vi "Quick Stacks - Image Multi Stacks.vi"(7 "Calling VI Ref":refnum<vi>) -> ()   [LabVIEW 2020]
uses:
  <vilib>/Utility/miscctls.llb/LVPointTypeDef.ctl
  Quick Stacks Type Defs/Quick Stack Marked Areas Actions.ctl
  Quick Stacks Type Defs/Quick Stacks Notifier Type.ctl
  Quick Stacks Type Defs/Quick Stack Actions.ctl
  Hardware Configuration/Hardware Configuration Controls/Device Function.ctl
  Hardware Configuration/Hardware Configuration Controls/Device Type.ctl
  Device Library/Stages/Stages Controls/Stage Actions.ctl
  Quick Stacks Type Defs/Quick Stacks Multi Stack Meta Data.ctl
  Device Library/Microscopes/Polymorphic Microscope Messenger/Get Obj Z Pos.vi
  Device Library/Microscopes/Polymorphic Microscope Messenger/Set Obj Z Pos.vi
panel:
  out "Current Delay Time (s)":dbl=1.0 format="%.1f"
  out "Current Cycle":u16=1 min=1
  out "XY Positions":cluster{dbl[], dbl[]}[](graph)
  in  "Cycle Delay (s)":u32
  in  "Number of Cycles":u16=1 min=1
  in  "Capture":bool
  in  "Clear All":bool
  in  "Clear Selected":bool
  in  "Mark Point":bool
  in  "Marked Positions":i32(listbox)
  in  "Quit":bool
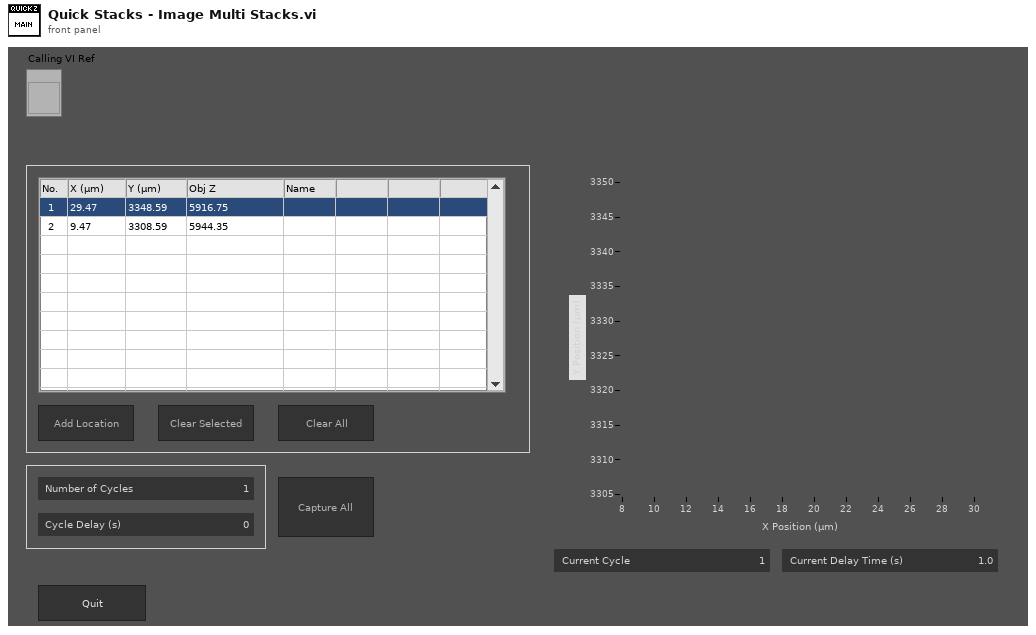
[diagram p1: front panel]
types:
  T1 = typedef "Quick Stacks Notifier Type.ctl" = cluster{"Actions":T2, "Start Z (µm)":dbl, "End Z (µm)":dbl, "Z Size (µm)":dbl, "Num of Steps":u16, "Frames per Step":u16, "Cycle Delay (s)":u32, "Num of Cycles":u16, "Save Path":path, "Running?":bool, "Save File Refs":refnum<file>[]}
  T2 = typedef "Quick Stack Actions.ctl" = enum16{"Idle", "Update Range", "Start Acquisition", "Initial C Step", "Open File", "Close File", "Start Camera", "Stop Camera", "Wait New Frame", "Laser On", "Laser Off", "Get Image", "Step Z", "Move to Z Start", "Step Color", "Check Cycle", "Abort", "Exit Loop", "Quit"}
  T3 = typedef "Quick Stack Marked Areas Actions.ctl" = enum16{"Add Position", "Update File Name", "Remove Position", "Start Capture", "Move to Position", "Write Meta Data", "Capture", "Switch", "Delay", "Reset Path", "Clear All", "Abort", "Exit Loop", "Quit"}
  T4 = enum16{"Always On", "Always Off", "Off While Running"}
  T5 = typedef "LVPointTypeDef.ctl" = cluster{"Horizontal":i16, "Vertical":i16}
  T6 = typedef "Device Function.ctl" = enum16{"Primary", "Secondary", "Overview", "Wide Field Drift Correction", "642 nm Excitation", "560 nm Excitation", "940 nm Excitation", "546 nm Excitation", "488 nm Excitation", "405 nm Excitation", "Objective Drift Correction", "4Pi Objective Lock", "Objective XY", "Objective Z", "Sample XY", "Sample Coarse Z", "Sample Z", "4Pi Lower", "4Pi Upper", "Mojo", "Adj Cavity", "Line Scanning", "Alert"}
  T7 = typedef "Device Type.ctl" = enum16{"AOTF", "Camera", "Deformable Mirror", "Laser", "Microscope Base", "Shutter", "Stage", "Waveform", "FPGA", "Email", "Filter Wheel", "Spinning Disk"}
  T8 = typedef "Stage Actions.ctl" = enum16{"Get Position", "MVR", "MOVE", "HALT", "ONTARGET", "ERROR", "REFERENCE", "INIT", "VELOCITY", "STATUS", "EXIT", "HOME", "ZEROPOS", "NANOPOS", "ANALOG", "QUIT"}
  T9 = typedef "Quick Stacks Multi Stack Meta Data.ctl" = cluster{"Start Z (µm)":dbl, "End Z (µm)":dbl, "Z Size (µm)":dbl, "Num of Steps":u16, "Frames per Step":u16, "Cycle Delay (s)":u32, "Num of Cycles":u16}
  T10 = enum32{"Invalid", "Standard", "Closed", "Hidden", "Minimized", "Maximized"}
  T11 = enum8{"Enabled", "Disabled", "Disabled and Grayed Out"}
  T12 = typedef "LVRectTypeDef.ctl" = cluster{"Left":i16, "Top":i16, "Right":i16, "Bottom":i16}
  T13 = typedef "LVBoundsTypeDef.ctl" = cluster{"Width":u32, "Height":u32}
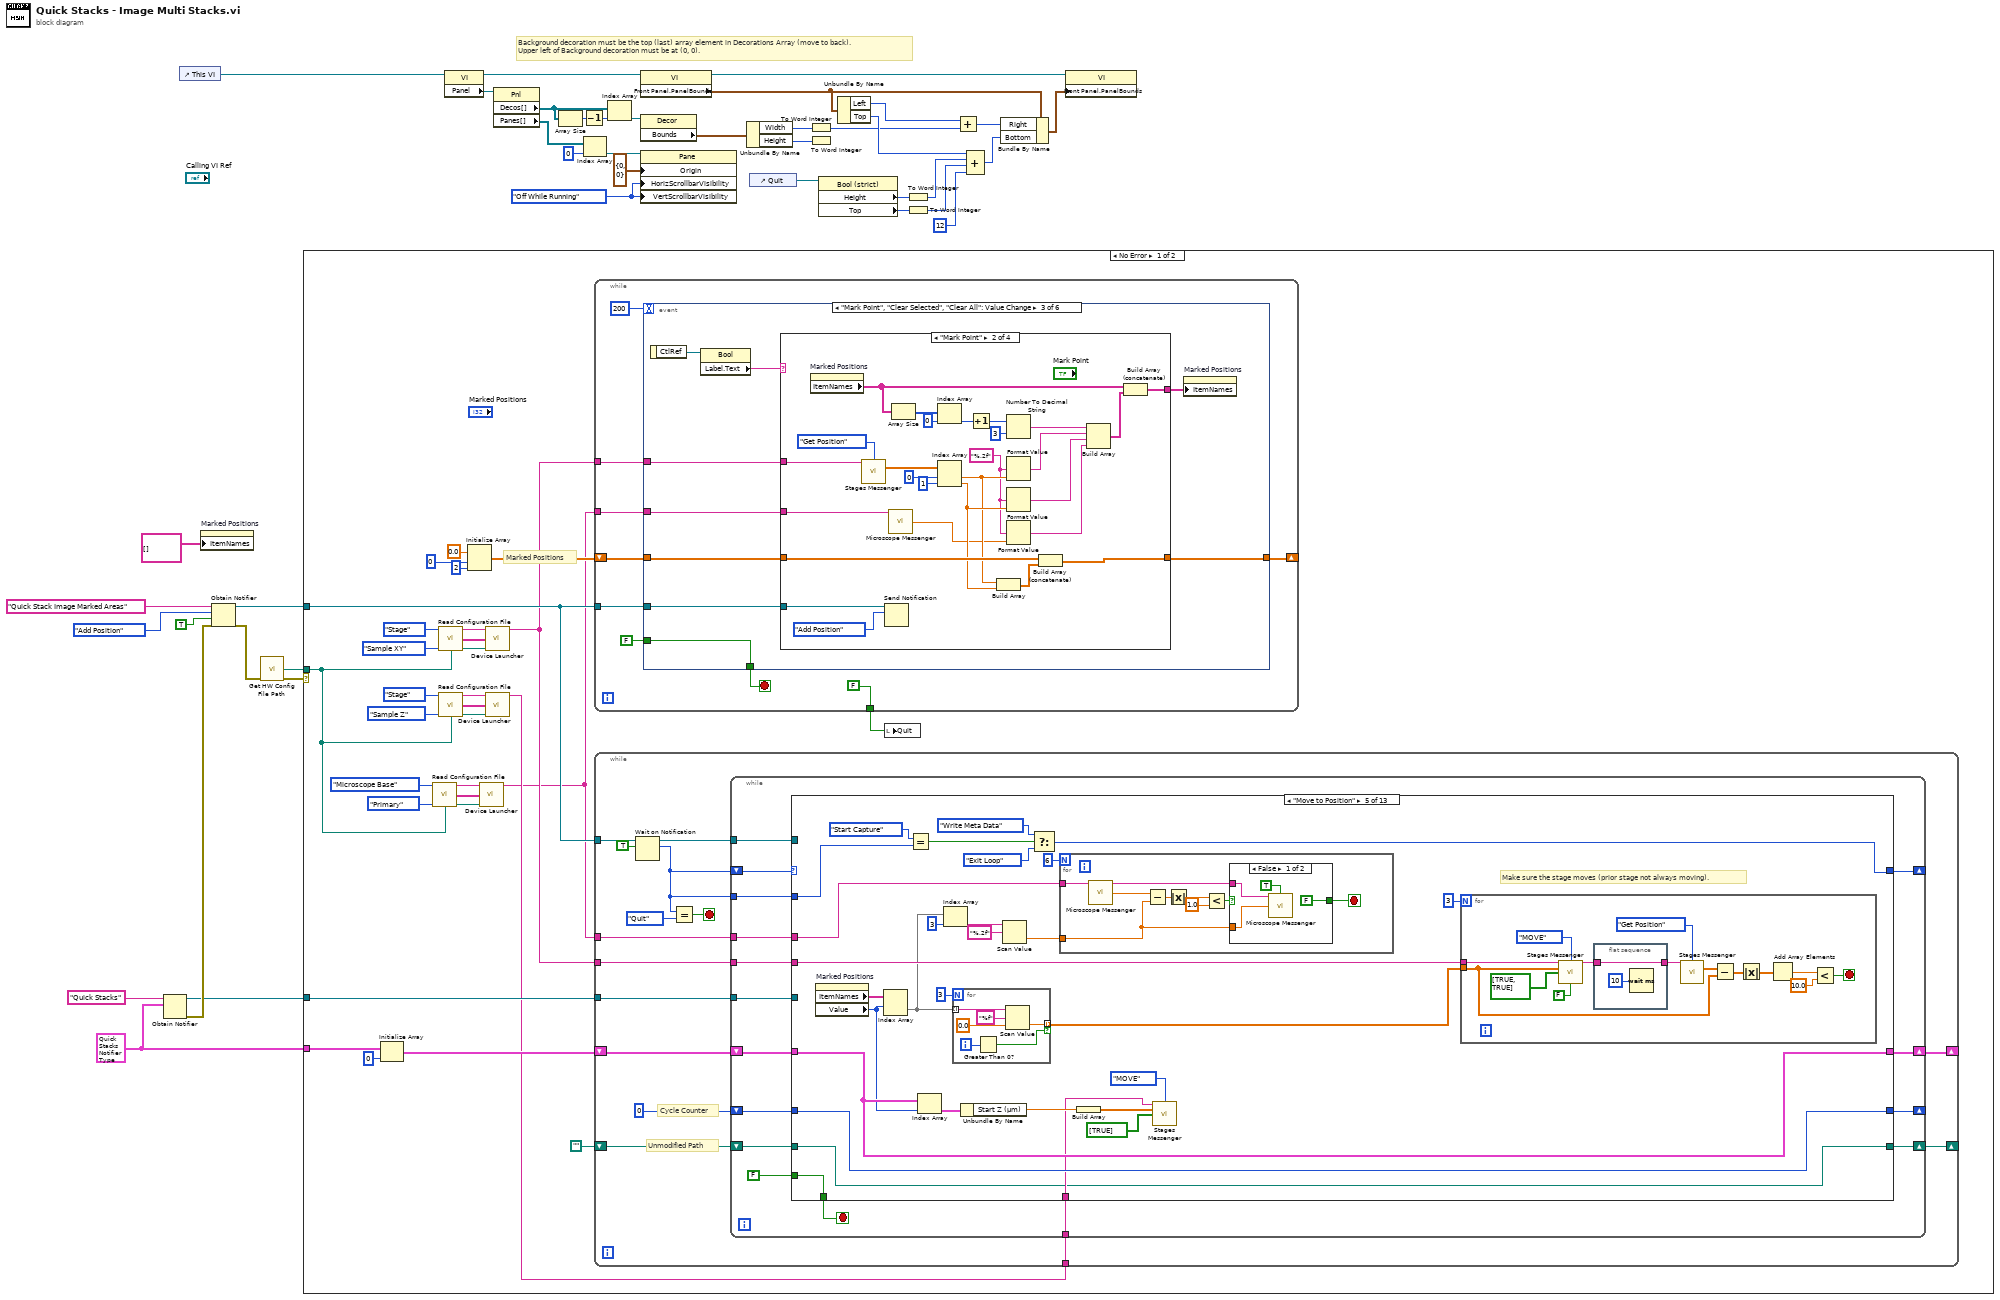
[diagram p0: block diagram]
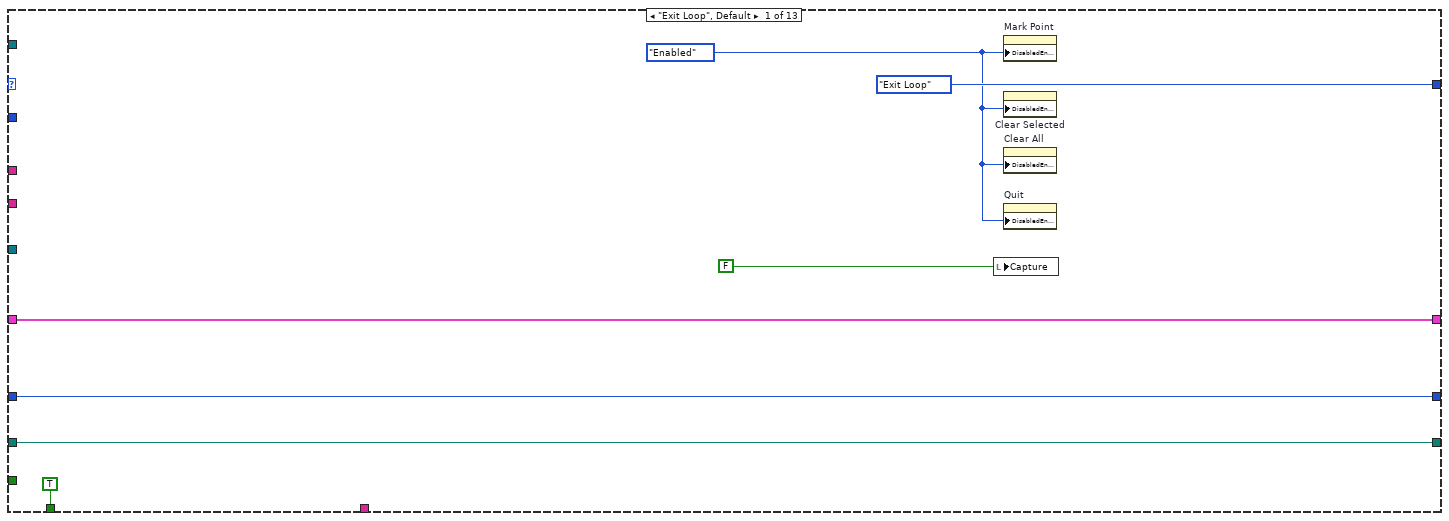
[diagram p2: hidden frame]
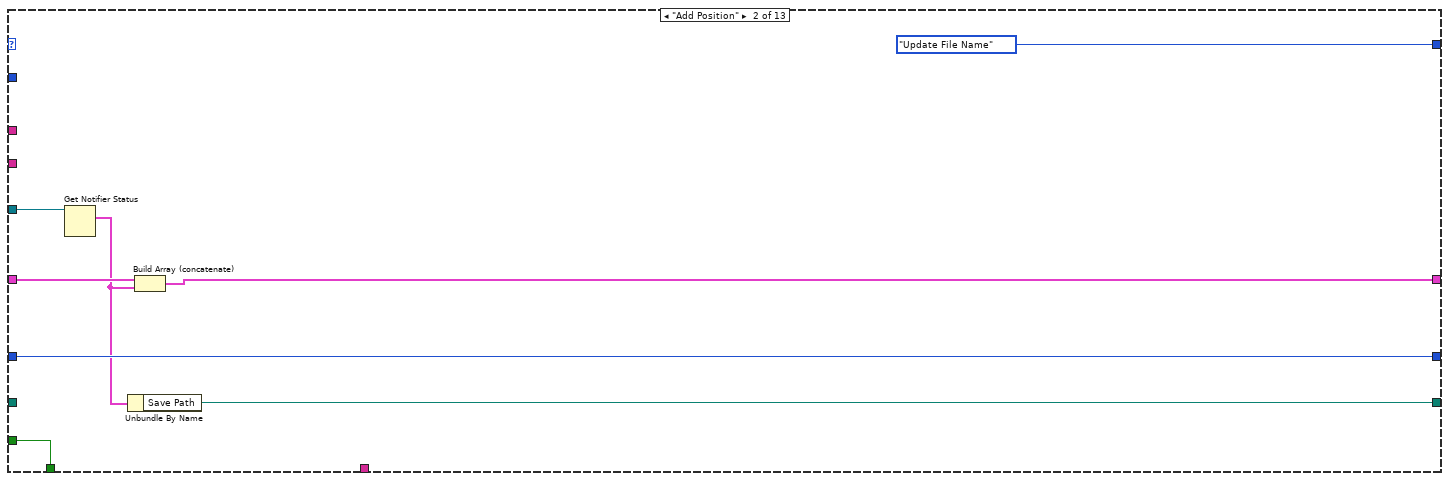
[diagram p3: hidden frame]
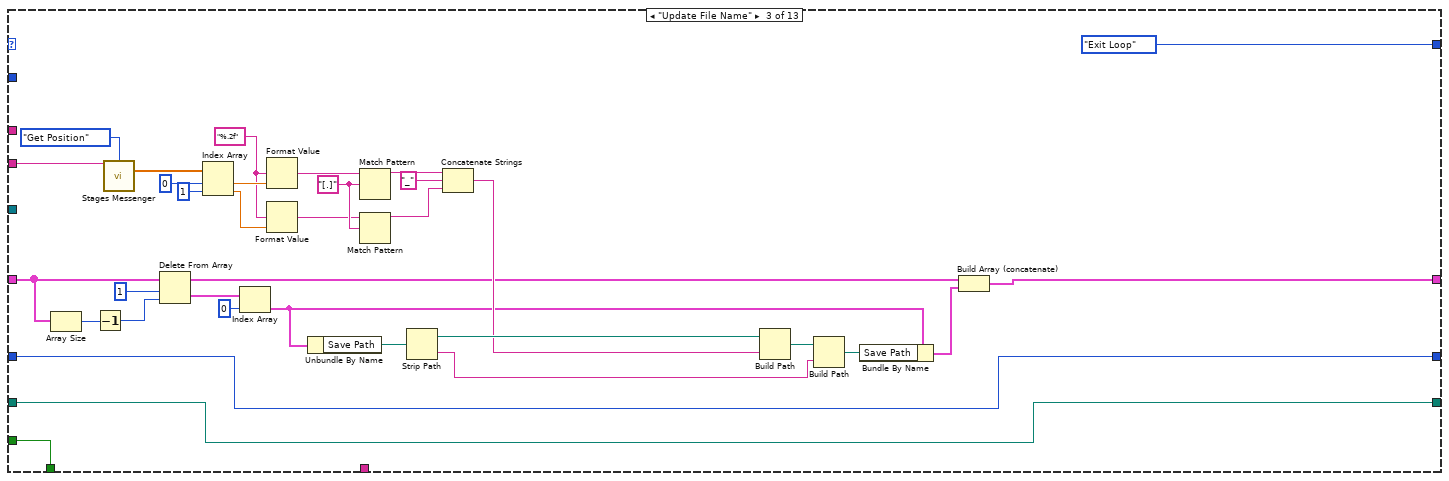
[diagram p4: hidden frame]
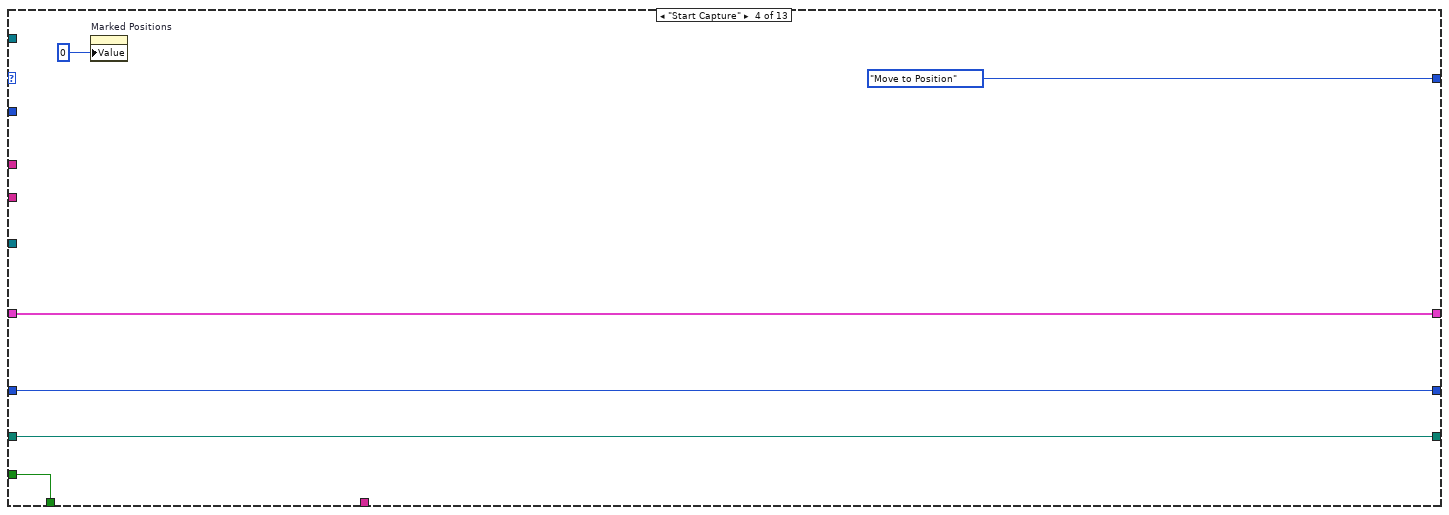
[diagram p5: hidden frame]
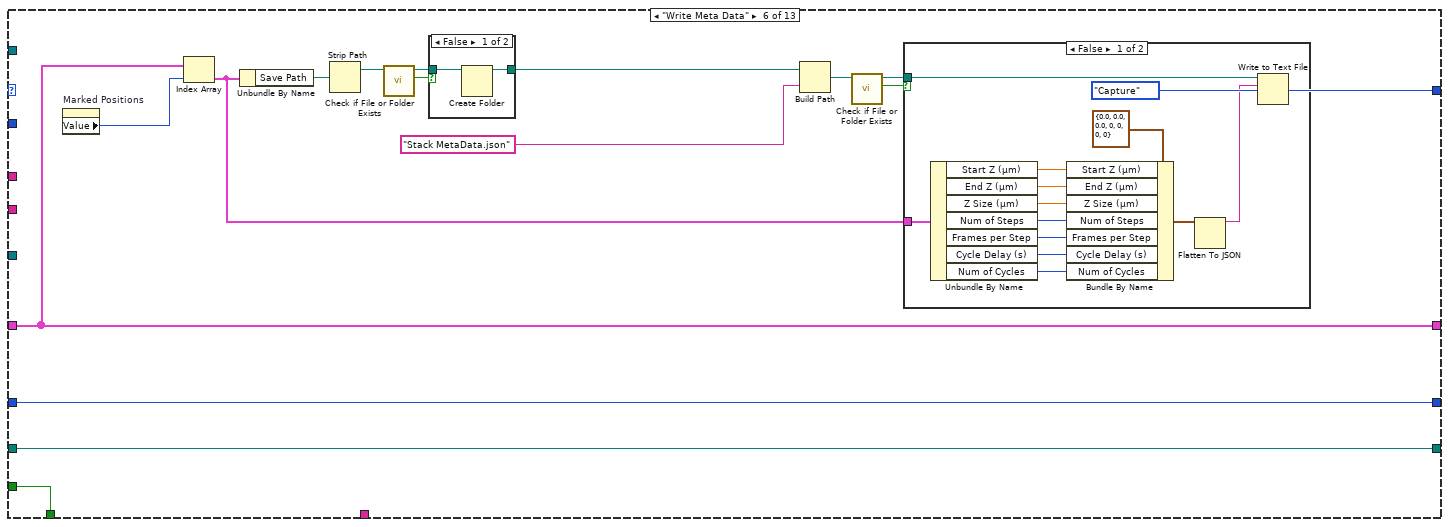
[diagram p7: hidden frame]
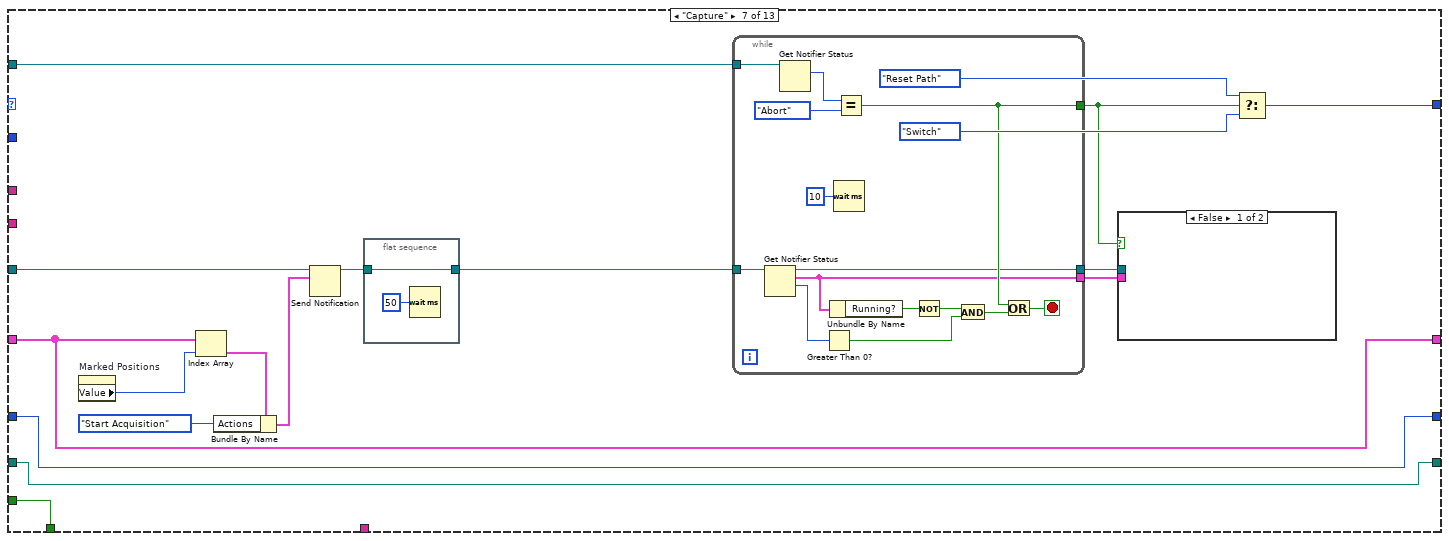
[diagram p10: hidden frame]
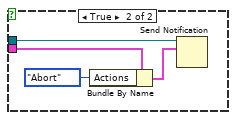
[diagram p11: hidden frame]
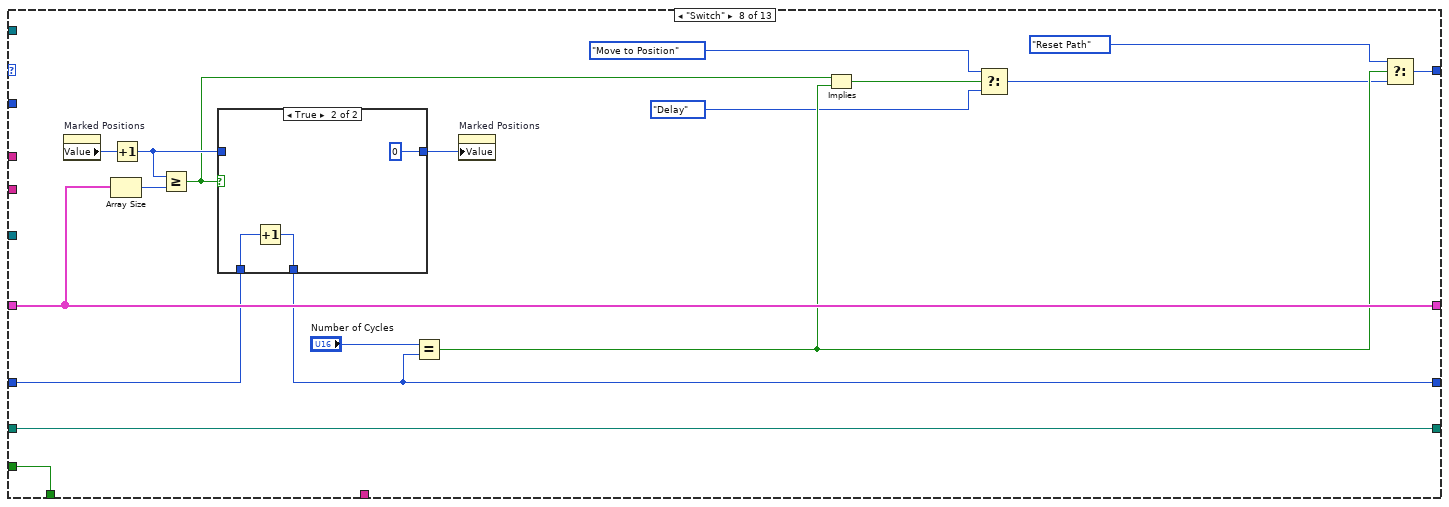
[diagram p12: hidden frame]
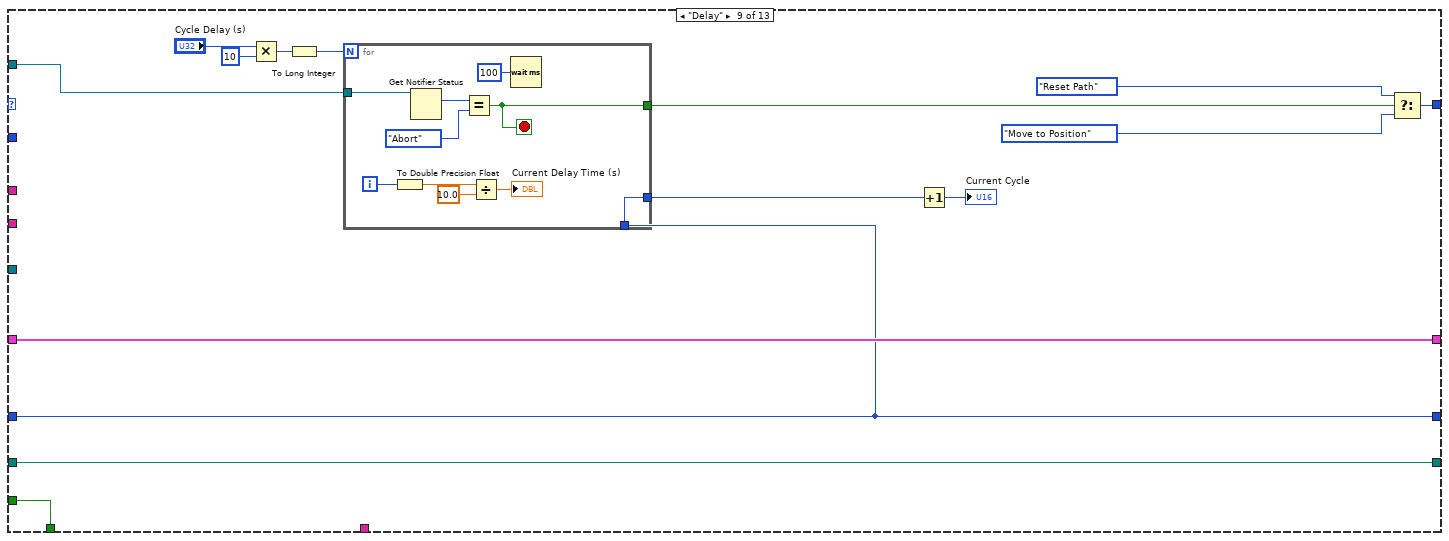
[diagram p14: hidden frame]
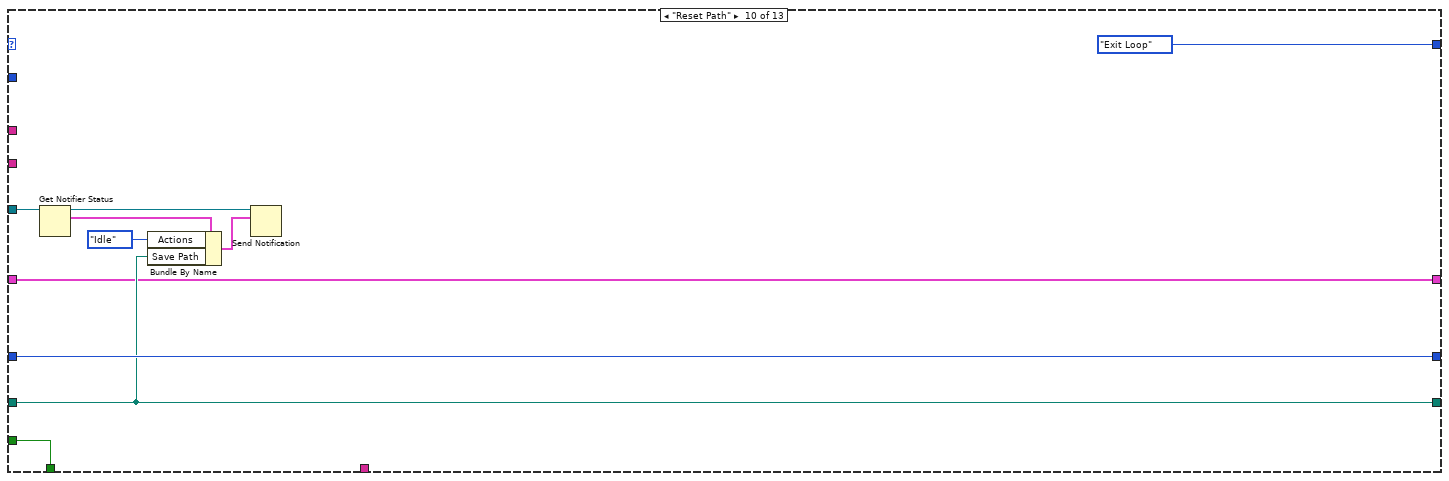
[diagram p15: hidden frame]
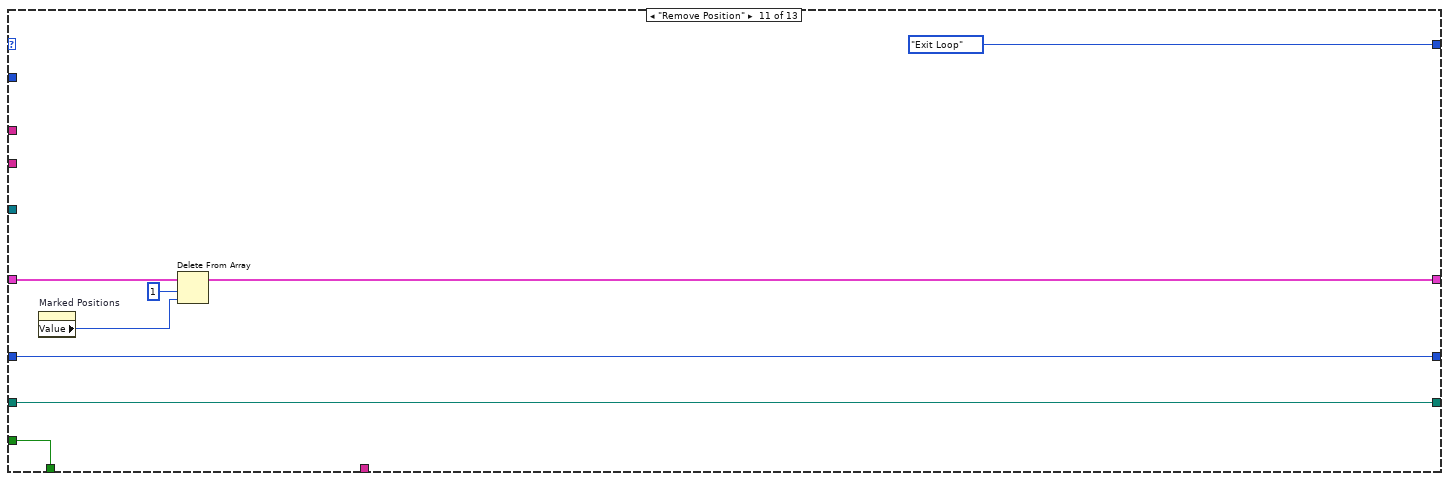
[diagram p16: hidden frame]
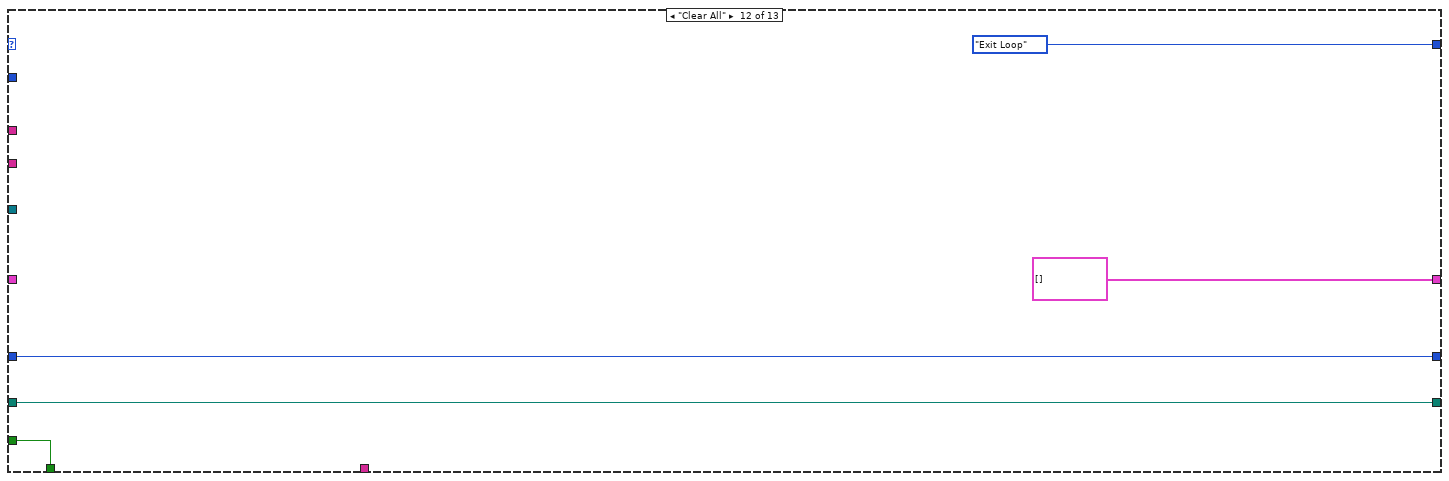
[diagram p17: hidden frame]
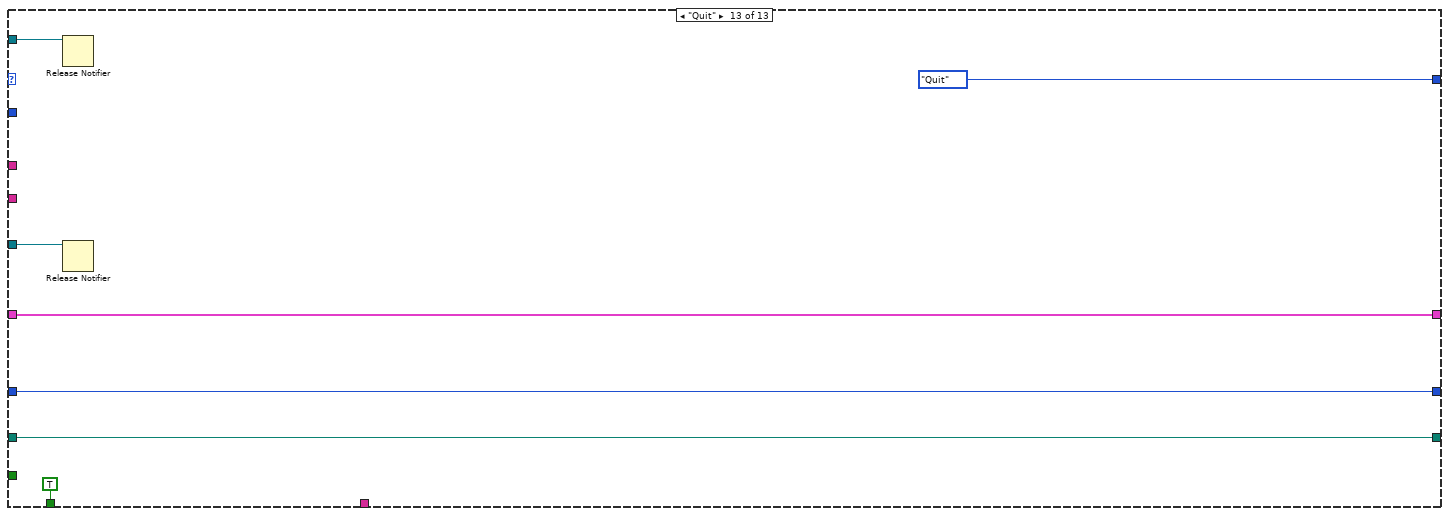
[diagram p18: hidden frame]
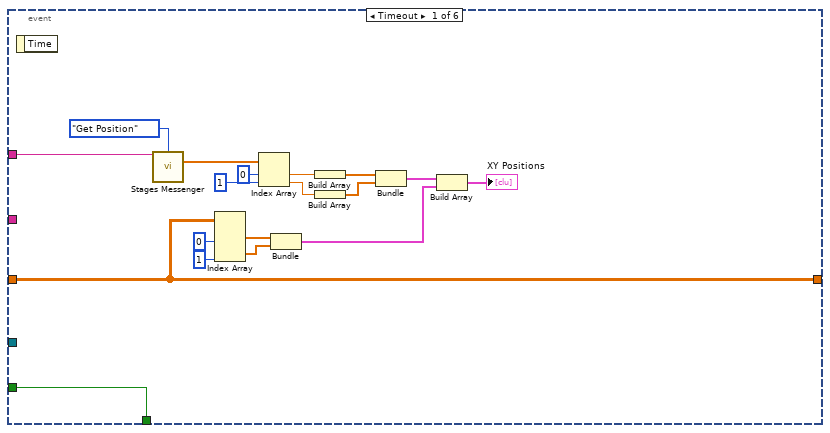
[diagram p19: hidden frame]
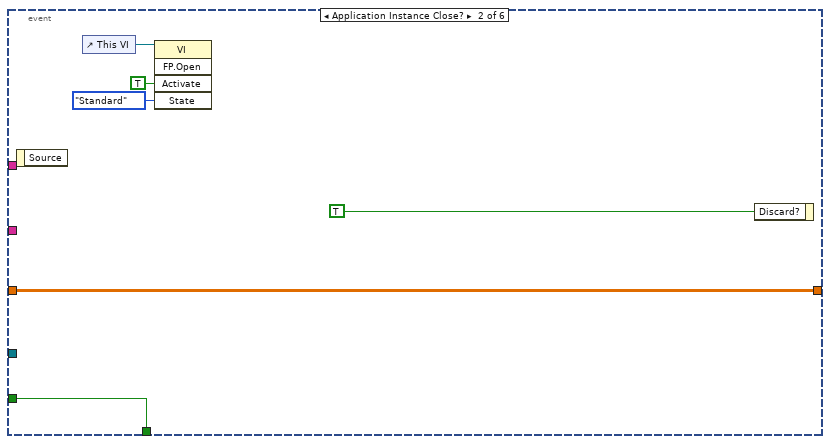
[diagram p20: hidden frame]
diagram:
  w1 = T1 {"Actions"=enum."Idle", "Start Z (µm)"=0.0, "End Z (µm)"=0.0, "Z Size (µm)"=0.0, "Num of Steps"=0, "Frames per Step"=0, "Cycle Delay (s)"=0, "Num of Cycles"=0, "Save Path"=path "", "Running?"=FALSE, "Save File Refs"=[]} ("Stack Parameters")
  w22 = T4."Off While Running" ("Vertical Scrollbar Visibility")
  # "Background decoration must be the top (last) array element in Decorations Array (move to back).\nUpper left of Background decoration must be at (0, 0)."
  n1 = Obtain Notifier(name (unnamed)="Quick Stacks", notification data type=w1) -> (notifier out=w2:refnum<notifier>, error out=w3:errorcluster)  [unwired: 2 in, 1 out]
  n2 = control-ref of="This VI"() -> (w14:refnum<vi>)
  n3 = property on="Marked Positions" class="MCListbox (strict)"("ItemNames"=string[][] [] ("Item Names")) -> ()  [unwired: 2 in, 2 out]
  n4 = Obtain Notifier(name (unnamed)="Quick Stack Image Marked Areas", notification data type=Quick_Stack_Marked_Areas_Actions."Add Position" ("Actions"), create if not found? (T)=TRUE, error in (no error)=w3) -> (notifier out=w7:refnum<notifier>, error out=w8:errorcluster)  [unwired: 1 out]
  n5 = call "Get HW Config File Path.vi"("Error"=w8) -> ("File Path"=w40:path, "Error"=w41:errorcluster)  [unwired: 13 in]
  n6 = case shown="No Error" w41 {
    tunnel: w40 -> [w43 _]
    tunnel: w7 -> [w65 _]
    tunnel: w2 -> [w63 _]
    tunnel: w1 -> [w62 _]
    frame No Error {
      # "Marked Positions"
      n7 = Initialize Array(w62, 0 ("dimension size")) -> (w60:T1[])
      n8 = call "Read Configuration File.vi"("Device Type"=Device_Type."Microscope Base", "Device Function"=Device_Function."Primary", "Config File Path"=w43) -> ("Unique Notifier Name"=w46:string, "Device Ports/IDs/Channels"=w48:string[], "Device Engine Path"=w47:path)  [unwired: 9 in, 1 out]
      n9 = call "Read Configuration File.vi"("Device Type"=Device_Type."Stage", "Device Function"=Device_Function."Sample XY", "Config File Path"=w43) -> ("Unique Notifier Name"=w69:string, "Device Ports/IDs/Channels"=w71:string[], "Device Engine Path"=w70:path)  [unwired: 9 in, 1 out]
      n10 = call "Read Configuration File.vi"("Device Type"=Device_Type."Stage", "Device Function"=Device_Function."Sample Z", "Config File Path"=w43) -> ("Unique Notifier Name"=w53:string, "Device Ports/IDs/Channels"=w51:string[], "Device Engine Path"=w52:path)  [unwired: 9 in, 1 out]
      n11 = Initialize Array(0.0 ("element"), 0 ("dimension size"), 2 ("dimension size")) -> (w58:dbl[][])
      n12 = call "Device Launcher.vi"("Notifier Name"=w46, "Device Ports/IDs/Channels"=w48, "Device Engine Path"=w47) -> ("Notifier Name"=w42:string)  [unwired: 11 in, 1 out]
      n13 = call "Device Launcher.vi"("Notifier Name"=w69, "Device Ports/IDs/Channels"=w71, "Device Engine Path"=w70) -> ("Notifier Name"=w64:string)  [unwired: 11 in, 1 out]
      n14 = call "Device Launcher.vi"("Notifier Name"=w53, "Device Ports/IDs/Channels"=w51, "Device Engine Path"=w52) -> ("Notifier Name"=w50:string)  [unwired: 11 in, 1 out]
      n15 = while {
        tunnel: [FALSE] -> w66
        tunnel: w64 -> [w374]
        tunnel: w65 -> [w373]
        shift-right: [w371] -> _
        shift-left: w58 -> [w372]
        tunnel: w42 -> [w370]
        stop <- w376 stop-if-true
        n16 = event shown="[2] \"Mark Point\", \"Clear Selected\", \"Clear All\": Value Change" {
          selector: _ -> [_ _ _ _ _ _]
          dyn-events: _ -> [_ _ _ _ _ _]
          timeout: 200 -> [_ _ _ _ _ _]
          tunnel: FALSE -> [w396 w401 w411 w466 w476 _]
          tunnel: [w396 w401 w411 w466 w476 w480] -> w376
          tunnel: w374 -> [w394 _ w408 _ _ _]
          tunnel: w373 -> [_ _ w406 w465 w475 w479]
          tunnel: w372 -> [w386 w397 w405 w463 w467 w477]
          tunnel: [w386 w397 w404 w463 w467 w477] -> w371
          tunnel: w370 -> [_ _ w403 _ _ _]
          event Timeout {
            n17 = event-data() -> ()  [unwired: 1 in, 1 out]
            n18 = call "Stages Messenger.vi"("Stage Notifier Name"=w394, "Actions"=Stage_Actions."Get Position") -> ("Positions"=w393:dbl[])  [unwired: 10 in, 3 out]
            n19 = Index Array(array=w386, index (col) #1=0 ("disabled index (col)"), index (col) #2=1 ("index (col)")) -> (element #1=w383:dbl[], element #2=w382:dbl[])  [unwired: 2 in]
            n20 = Index Array(array=w393, index #1=0 ("index"), index #2=1 ("index")) -> (element #1=w390:dbl, element #2=w389:dbl)
            n21 = Bundle(w383, w382) -> (w380:cluster{dbl[], dbl[]})  [unwired: 1 in]
            n22 = Build Array(w390) -> (w388:dbl[])
            n23 = Build Array(w389) -> (w387:dbl[])
            n24 = Bundle(w388, w387) -> (w381:cluster{dbl[], dbl[]})  [unwired: 1 in]
            n25 = Build Array(w381, w380) -> (→"XY Positions":cluster{dbl[], dbl[]}[])
          }
          event Application Instance Close? {
            n26 = event-data() -> ()  [unwired: 1 in, 1 out]
            n27 = control-ref of="This VI"() -> (w398:refnum<vi>)
            n28 = invoke class="VI" method="FP.Open"(reference=w398, "Activate"=TRUE ("Activate?"), "State"=T10."Standard") -> ()  [unwired: 2 in, 5 out]
            n29 = event-data("Discard?"=TRUE) -> ()  [unwired: 1 in, 1 out]
          }
          event "Mark Point", "Clear Selected", "Clear All": Value Change {
            n30 = event-data() -> ("CtlRef"=w410:refnum<vi>)  [unwired: 1 in]
            n31 = property class="Bool"(reference=w410) -> ("Label.Text"=w407:string)  [unwired: 1 in, 2 out]
            n32 = case shown="\"Mark Point\"" w407 {
              tunnel: [w415 w431 w452 string[][] []] -> w409
              tunnel: w408 -> [_ w429 _ _]
              tunnel: w406 -> [w414 w428 w450 w461]
              tunnel: w405 -> [w412 w426 w446 _]
              tunnel: [w412 w422 w444 w456] -> w404
              tunnel: w403 -> [_ w421 _ _]
              frame Default {
                n33 = Send Notification(notification=Quick_Stack_Marked_Areas_Actions."Exit Loop", notifier=w414) -> ()  [unwired: 1 in, 2 out]
                n34 = property on="Marked Positions" class="MCListbox (strict)"() -> ("ItemNames"=w415:string[][])  [unwired: 2 in, 2 out]
              }
              frame "Mark Point" {
                w419 = "%.2f" ("format string")
                n35 = property on="Marked Positions" class="MCListbox (strict)"() -> ("ItemNames"=w418:string[][])  [unwired: 2 in, 2 out]
                n36 = call "Stages Messenger.vi"("Stage Notifier Name"=w429, "Actions"=Stage_Actions."Get Position") -> ("Positions"=w430:dbl[])  [unwired: 10 in, 3 out]
                n37 = Send Notification(notification=Quick_Stack_Marked_Areas_Actions."Add Position", notifier=w428) -> ()  [unwired: 1 in, 2 out]
                n38 = call-poly "Microscope Messenger.vi"("Notifier Name In"=w421) -> ("Obj Z Pos"=w416:dbl)  [unwired: 12 in, 2 out]
                n39 = Array Size(array=w418) -> (size(s)=w437:i32[])
                n40 = Index Array(array=w437, index=0) -> (element=w435:i32)
                n41 = Index Array(array=w430, index #1=0 ("index"), index #2=1 ("index")) -> (element #1=w424:dbl, element #2=w425:dbl)
                n42 = Increment(x=w435) -> (x+1=w439:i32)
                n43 = Build Array(w424, w425) -> (w423:dbl[])
                n44 = Number To Decimal String(number=w439, width (-)=i16 3) -> (decimal integer string=w434:string)
                n45 = Format Value(format string=w419, value (0)=w424) -> (output string=w433:string)  [unwired: 1 in]
                n46 = Format Value(format string=w419, value (0)=w425) -> (output string=w420:string)  [unwired: 1 in]
                n47 = Format Value(format string=w419, value (0)=w416) -> (output string=w417:string)  [unwired: 1 in]
                n48 = Build Array (concatenate)(w426, w423) -> (w422:dbl[][])
                n49 = Build Array(w434, w433, w420, w417) -> (w432:string[])
                n50 = Build Array (concatenate)(w418, w432) -> (w431:string[][])
              }
              frame "Clear Selected" {
                n51 = Send Notification(notification=Quick_Stack_Marked_Areas_Actions."Remove Position", notifier=w450) -> (error out=w448:errorcluster)  [unwired: 1 in, 1 out]
                n52 = flat-sequence {
                  tunnel: w448 -> [w454]
                  tunnel: [w454] -> w447
                  frame #0 {
                    n53 = Wait (ms)(milliseconds to wait=u32 10) -> ()  [unwired: 1 out]
                  }
                }
                n54 = property on="Marked Positions" class="MCListbox (strict)"() -> ("ItemNames"=w453:string[][])  [unwired: 2 in, 2 out]
                n55 = property on="Marked Positions" class="MCListbox (strict)"(error in=w447) -> ("Value"=w445:i32)  [unwired: 1 in, 2 out]
                n56 = Delete From Array(array=w453, length=1, index (row)=w445) -> (array with subset deleted=w452:string[][])  [unwired: 1 in, 1 out]
                n57 = Delete From Array(array=w446, length=1, index (row)=w445) -> (array with subset deleted=w444:dbl[][])  [unwired: 1 in, 1 out]
              }
              frame "Clear All" {
                n58 = Send Notification(notification=Quick_Stack_Marked_Areas_Actions."Clear All", notifier=w461) -> ()  [unwired: 1 in, 2 out]
                n59 = Initialize Array(0.0 ("element"), 0 ("dimension size"), 2 ("dimension size")) -> (w456:dbl[][])
              }
            }
            n60 = property on="Marked Positions" class="MCListbox (strict)"("ItemNames"=w409) -> ()  [unwired: 2 in, 2 out]
          }
          event "Marked Positions": Double Click {
            n61 = event-data() -> ()  [unwired: 1 in, 1 out]
            n62 = Send Notification(notification=Quick_Stack_Marked_Areas_Actions."Move to Position", notifier=w465) -> ()  [unwired: 1 in, 2 out]
          }
          event "Capture": Value Change {
            n63 = event-data() -> ("NewVal"=w472:bool)  [unwired: 1 in]
            n64 = Select(t=Quick_Stack_Marked_Areas_Actions."Start Capture", s=w472, f=Quick_Stack_Marked_Areas_Actions."Abort" ("y")) -> (s? t:f=w473:T3)
            n65 = Select(t=T11."Disabled and Grayed Out" ("Disabled"), s=w472, f=T11."Enabled" ("Disabled")) -> (s? t:f=w469:T11)
            n66 = Send Notification(notification=w473, notifier=w475) -> ()  [unwired: 1 in, 2 out]
            n67 = property on="Mark Point" class="Bool"("DisabledEnum"=w469) -> ()  [unwired: 2 in, 2 out]
            n68 = property on="Clear Selected" class="Bool"("DisabledEnum"=w469) -> ()  [unwired: 2 in, 2 out]
            n69 = property on="Clear All" class="Bool"("DisabledEnum"=w469) -> ()  [unwired: 2 in, 2 out]
            n70 = property on="Quit" class="Bool (strict)"("DisabledEnum"=w469) -> ()  [unwired: 2 in, 2 out]
          }
          event "Quit": Value Change {
            n71 = event-data() -> ("NewVal"=w480:bool)  [unwired: 1 in]
            n72 = Send Notification(notification=Quick_Stack_Marked_Areas_Actions."Quit", notifier=w479) -> ()  [unwired: 1 in, 2 out]
          }
        }
      }
      n73 = while {
        tunnel: w65 -> [w86]
        tunnel: w64 -> [w80]
        tunnel: w63 -> [w79]
        shift-right: [w77] -> _
        shift-left: w60 -> [w78]
        tunnel: w50 -> [w75]
        shift-right: [w74] -> _
        shift-left: path "" -> [w73]
        tunnel: w42 -> [w72]
        stop <- w83 stop-if-true
        # "Unmodified Path"
        # "Cycle Counter"
        n74 = Wait on Notification(notifier=w86, ignore previous (F)=TRUE) -> (notifier out=w82:refnum<notifier>, notification=w81:T3)  [unwired: 2 in, 2 out]
        n75 = Equal?(x=w81, y=Quick_Stack_Marked_Areas_Actions."Quit") -> (x = y?=w83:bool)
        n76 = while {
          shift-right: [w98] -> _
          shift-left: w81 -> [w101]
          tunnel: w82 -> [w102]
          tunnel: w81 -> [w97]
          tunnel: w80 -> [w96]
          tunnel: w79 -> [w95]
          shift-right: [w93] -> w77
          shift-left: w78 -> [w94]
          shift-right: [w91] -> _
          shift-left: u16 0 -> [w92]
          tunnel: w75 -> [w90]
          shift-right: [w89] -> w74
          shift-left: w73 -> [w88]
          tunnel: w72 -> [w87]
          stop <- w99 stop-if-true
          n77 = case shown="\"Move to Position\"" w101 {
            tunnel: w102 -> [_ _ _ _ _ _ w270 _ w320 _ _ _ w367]
            tunnel: [TRUE w117 w151 w157 w186 w237 w271 w309 w329 w348 w356 w361 TRUE] -> w99
            tunnel: FALSE -> [_ w117 w151 w157 w186 w237 w271 w309 w329 w348 w356 w361 _]
            tunnel: [Quick_Stack_Marked_Areas_Actions."Exit Loop" ("y") Quick_Stack_Marked_Areas_Actions."Update File Name" ("y") Quick_Stack_Marked_Areas_Actions."Exit Loop" ("y") Quick_Stack_Marked_Areas_Actions."Move to Position" ("y") w180 Quick_Stack_Marked_Areas_Actions."Capture" ("y") w268 w305 w321 Quick_Stack_Marked_Areas_Actions."Exit Loop" ("y") Quick_Stack_Marked_Areas_Actions."Exit Loop" ("y") Quick_Stack_Marked_Areas_Actions."Exit Loop" ("y") Quick_Stack_Marked_Areas_Actions."Quit" ("y")] -> w98
            tunnel: w97 -> [_ _ _ _ w183 _ _ _ _ _ _ _ _]
            tunnel: w96 -> [_ _ w131 _ w178 _ _ _ _ _ _ _ _]
            tunnel: w95 -> [_ w115 _ _ _ _ w263 _ _ w346 _ _ w366]
            tunnel: w94 -> [w105 w114 w140 w154 w174 w225 w260 w304 w328 w340 w353 _ w365]
            tunnel: [w105 w113 w122 w154 w174 w225 w260 w304 w328 w340 w352 T1[] [] w365] -> w93
            tunnel: w92 -> [w104 w112 w147 w153 w175 w236 w256 w301 w318 w349 w351 w359 w364]
            tunnel: [w104 w112 w147 w153 w175 w236 w256 w299 w318 w349 w351 w359 w364] -> w91
            tunnel: w90 -> [_ _ _ _ w167 _ _ _ _ _ _ _ _]
            tunnel: [w103 w110 w118 w152 w166 w223 w254 w292 w315 w341 w350 w358 w363] -> w89
            tunnel: w88 -> [w103 _ w118 w152 w166 w223 w254 w292 w315 w341 w350 w358 w363]
            tunnel: w87 -> [_ _ _ _ w160 _ _ _ _ _ _ _ _]
            frame "Exit Loop", Default {
              w107 = T11."Enabled" ("Disabled")
              n78 = local write "Capture"(FALSE ("Capture")) -> ()
              n79 = property on="Mark Point" class="Bool"("DisabledEnum"=w107) -> ()  [unwired: 2 in, 2 out]
              n80 = property on="Clear Selected" class="Bool"("DisabledEnum"=w107) -> ()  [unwired: 2 in, 2 out]
              n81 = property on="Clear All" class="Bool"("DisabledEnum"=w107) -> ()  [unwired: 2 in, 2 out]
              n82 = property on="Quit" class="Bool (strict)"("DisabledEnum"=w107) -> ()  [unwired: 2 in, 2 out]
            }
            frame "Add Position" {
              n83 = Get Notifier Status(notifier=w115) -> (current notification=w111:T1)  [unwired: 1 in, 4 out]
              n84 = Unbundle By Name(w111) -> ("Save Path"=w110:path)
              n85 = Build Array (concatenate)(w114, w111) -> (w113:T1[])
            }
            frame "Update File Name" {
              w132 = "%.2f" ("format string")
              w146 = "[.]" ("regular expression")
              n86 = Array Size(array=w140) -> (size(s)=w141:i32)
              n87 = Decrement(x=w141) -> (x-1=w138:i32)
              n88 = call "Stages Messenger.vi"("Stage Notifier Name"=w131, "Actions"=Stage_Actions."Get Position") -> ("Positions"=w133:dbl[])  [unwired: 10 in, 3 out]
              n89 = Delete From Array(array=w140, length=1, index=w138) -> (deleted portion=w126:T1[], array with subset deleted=w127:T1[])
              n90 = Index Array(array=w133, index #1=0 ("index"), index #2=1 ("index")) -> (element #1=w135:dbl, element #2=w134:dbl)
              n91 = Index Array(array=w126, index=0) -> (element=w124:T1)
              n92 = Format Value(format string=w132, value (0)=w135) -> (output string=w129:string)  [unwired: 1 in]
              n93 = Format Value(format string=w132, value (0)=w134) -> (output string=w128:string)  [unwired: 1 in]
              n94 = Unbundle By Name(w124) -> ("Save Path"=w150:path)
              n95 = Match Pattern(string=w129, regular expression=w146) -> (before substring=w145:string)  [unwired: 1 in, 3 out]
              n96 = Match Pattern(string=w128, regular expression=w146) -> (before substring=w144:string)  [unwired: 1 in, 3 out]
              n97 = Strip Path(path=w150) -> (stripped path=w149:path, name=w120:string)
              n98 = Concatenate Strings(w145, "_" ("string"), w144) -> (w142:string)
              n99 = Build Path(base path=w149, name or relative path=w142) -> (appended path=w121:path)
              n100 = Build Path(base path=w121, name or relative path=w120) -> (appended path=w119:path)
              n101 = Bundle By Name(cluster=w124, "Save Path"=w119) -> (w123:T1)
              n102 = Build Array (concatenate)(w127, w123) -> (w122:T1[])
            }
            frame "Start Capture" {
              n103 = property on="Marked Positions" class="MCListbox (strict)"("Value"=0 ("Focus Row")) -> ()  [unwired: 2 in, 2 out]
            }
            frame "Move to Position" {
              # "Make sure the stage moves (prior stage not always moving)."
              n104 = property on="Marked Positions" class="MCListbox (strict)"() -> ("ItemNames"=w179:string[][], "Value"=w173:i32)  [unwired: 2 in, 2 out]
              n105 = Index Array(array=w179, index (row)=w173) -> (element=w164:string[])  [unwired: 1 in]
              n106 = Equal?(x=Quick_Stack_Marked_Areas_Actions."Start Capture" ("y"), y=w183) -> (x = y?=w185:bool)
              n107 = Index Array(array=w174, index=w173) -> (element=w172:T1)
              n108 = Index Array(array=w164, index=3) -> (element=w161:string)
              n109 = for {
                N: 3 -> [_]
                tunnel: w164 -> [w220] mode=indexing
                tunnel: [w219] -> w177 mode=indexing if=w217
                i -> [w218]
                n110 = Greater Than 0?(x=w218) -> (x > 0?=w217:bool)
                n111 = Scan Value(string=w220, format string="%f", default (0 dbl)=0.0) -> (value=w219:dbl)  [unwired: 1 out]
              }
              n112 = Unbundle By Name(w172) -> ("Start Z (µm)"=w170:dbl)
              n113 = Scan Value(string=w161, format string="%.2f") -> (value=w159:dbl)  [unwired: 1 in, 1 out]
              n114 = Select(t=Quick_Stack_Marked_Areas_Actions."Write Meta Data", s=w185, f=Quick_Stack_Marked_Areas_Actions."Exit Loop" ("y")) -> (s? t:f=w180:T3)
              n115 = for {
                N: 6 -> [_]
                tunnel: w160 -> [w195]
                tunnel: w159 -> [w188]
                stop <- w187 stop-if-true
                n116 = call-poly "Microscope Messenger.vi"("Notifier Name In"=w195) -> ("Notifier Name Out"=w192:string, "Obj Z Pos"=w194:dbl)  [unwired: 12 in, 1 out]
                n117 = Subtract(x=w194, y=w188) -> (x-y=w190:dbl)
                n118 = Absolute Value(x=w190) -> (abs(x)=w189:dbl)
                n119 = Less?(x=w189, y=1.0) -> (x < y?=w191:bool)
                n120 = case shown="False" w191 {
                  selector: w191 -> [_ w200]
                  tunnel: w192 -> [w198 _]
                  tunnel: w188 -> [w197 _]
                  tunnel: [FALSE w200] -> w187
                  frame False {
                    n121 = call-poly "Microscope Messenger.vi"("Notifier Name In"=w198, "Wait to Finish"=TRUE, "Obj Z Pos (um)"=w197) -> ()  [unwired: 11 in, 2 out]
                  }
                  frame True {
                  }
                }
              }
              n122 = Build Array(w170) -> (w169:dbl[])
              n123 = call "Stages Messenger.vi"("Stage Notifier Name"=w167, "Actions"=Stage_Actions."MOVE", "Setpoint"=w169, "Axis"=bool[] [TRUE]) -> ()  [unwired: 8 in, 4 out]
              n124 = for {
                N: 3 -> [_]
                tunnel: w178 -> [w211]
                tunnel: w177 -> [w206]
                stop <- w201 stop-if-true
                n125 = call "Stages Messenger.vi"("Stage Notifier Name"=w211, "Actions"=Stage_Actions."MOVE", "Setpoint"=w206, "Axis"=bool[] [TRUE, TRUE], "Exit While Busy?"=FALSE ("Wait for On Target? (F)")) -> ("Stage Notifier Name (Dup)"=w210:string)  [unwired: 7 in, 3 out]
                n126 = flat-sequence {
                  tunnel: w210 -> [w215]
                  tunnel: [w215] -> w208
                  frame #0 {
                    n127 = Wait (ms)(milliseconds to wait=u32 10) -> ()  [unwired: 1 out]
                  }
                }
                n128 = call "Stages Messenger.vi"("Stage Notifier Name"=w208, "Actions"=Stage_Actions."Get Position") -> ("Positions"=w207:dbl[])  [unwired: 10 in, 3 out]
                n129 = Subtract(x=w207, y=w206) -> (x-y=w205:dbl[])
                n130 = Absolute Value(x=w205) -> (abs(x)=w204:dbl[])
                n131 = Add Array Elements(numeric array=w204) -> (sum=w203:dbl)
                n132 = Less?(x=w203, y=10.0) -> (x < y?=w201:bool)
              }
            }
            frame "Write Meta Data" {
              n133 = property on="Marked Positions" class="MCListbox (strict)"() -> ("Value"=w235:i32)  [unwired: 2 in, 2 out]
              n134 = Index Array(array=w225, index=w235) -> (element=w224:T1)
              n135 = Unbundle By Name(w224) -> ("Save Path"=w234:path)
              n136 = Strip Path(path=w234) -> (stripped path=w229:path)  [unwired: 1 out]
              n137 = call <vilib>:"Check if File or Folder Exists.vi"("path"=w229) -> ("file or folder exists?"=w228:bool, "dup path"=w227:path)  [unwired: 8 in, 1 out]
              n138 = case shown="False" w228 {
                tunnel: w227 -> [w240 w241]
                tunnel: [w239 w241] -> w226
                frame False {
                  n139 = Create Folder(path (use dialog)=w240) -> (created path=w239:path)  [unwired: 2 in, 2 out]
                }
                frame True {
                }
              }
              n140 = Build Path(base path=w226, name or relative path="Stack MetaData.json") -> (appended path=w232:path)
              n141 = call <vilib>:"Check if File or Folder Exists.vi"("path"=w232) -> ("file or folder exists?"=w231:bool, "dup path"=w230:path)  [unwired: 8 in, 1 out]
              n142 = case shown="False" w231 {
                tunnel: w230 -> [w253 _]
                tunnel: w224 -> [w244 _]
                frame False {
                  n143 = Unbundle By Name(w244) -> ("Start Z (µm)"=w246:dbl, "End Z (µm)"=w247:dbl, "Z Size (µm)"=w248:dbl, "Num of Steps"=w249:u16, "Frames per Step"=w250:u16, "Cycle Delay (s)"=w251:u32, "Num of Cycles"=w242:u16)
                  n144 = Bundle By Name(cluster=T9 {"Start Z (µm)"=0.0, "End Z (µm)"=0.0, "Z Size (µm)"=0.0, "Num of Steps"=0, "Frames per Step"=0, "Cycle Delay (s)"=0, "Num of Cycles"=0} ("Stack Parameters"), "Start Z (µm)"=w246, "End Z (µm)"=w247, "Z Size (µm)"=w248, "Num of Steps"=w249, "Frames per Step"=w250, "Cycle Delay (s)"=w251, "Num of Cycles"=w242) -> (w252:T9)
                  n145 = Flatten To JSON(anything=w252) -> (JSON string=w243:string)  [unwired: 2 in, 1 out]
                  n146 = Write to Text File(file (use dialog)=w253, text=w243) -> ()  [unwired: 2 in, 3 out]
                }
                frame True {
                }
              }
            }
            frame "Capture" {
              n147 = property on="Marked Positions" class="MCListbox (strict)"() -> ("Value"=w266:i32)  [unwired: 2 in, 2 out]
              n148 = Index Array(array=w260, index=w266) -> (element=w267:T1)
              n149 = Bundle By Name(cluster=w267, "Actions"=Quick_Stack_Actions."Start Acquisition") -> (w264:T1)
              n150 = Send Notification(notification=w264, notifier=w263) -> (notifier out=w262:refnum<notifier>)  [unwired: 1 in, 1 out]
              n151 = flat-sequence {
                tunnel: w262 -> [w277]
                tunnel: [w277] -> w261
                frame #0 {
                  n152 = Wait (ms)(milliseconds to wait=u32 50) -> ()  [unwired: 1 out]
                }
              }
              n153 = while {
                tunnel: w270 -> [w291]
                tunnel: [w289] -> w259
                tunnel: w261 -> [w286]
                tunnel: [w280] -> w258
                tunnel: [w279] -> w257
                stop <- w290 stop-if-true
                n154 = Get Notifier Status(notifier=w286) -> (notifier out=w280:refnum<notifier>, current notification=w279:T1, # waiting=w285:i32)  [unwired: 1 in, 2 out]
                n155 = Get Notifier Status(notifier=w291) -> (current notification=w278:T3)  [unwired: 1 in, 4 out]
                n156 = Greater Than 0?(x=w285) -> (x > 0?=w282:bool)
                n157 = Unbundle By Name(w279) -> ("Running?"=w284:bool)
                n158 = Wait (ms)(milliseconds to wait=u32 10) -> ()  [unwired: 1 out]
                n159 = Equal?(x=w278, y=Quick_Stack_Marked_Areas_Actions."Abort") -> (x = y?=w289:bool)
                n160 = Not(x=w284) -> (.not. x?=w283:bool)
                n161 = And(x=w283, y=w282) -> (x .and. y?=w281:bool)
                n162 = Or(x=w289, y=w281) -> (x .or. y?=w290:bool)
              }
              n163 = case shown="False" w259 {
                tunnel: w258 -> [_ w273]
                tunnel: w257 -> [_ w275]
                frame False {
                }
                frame True {
                  n164 = Bundle By Name(cluster=w275, "Actions"=Quick_Stack_Actions."Abort") -> (w272:T1)
                  n165 = Send Notification(notification=w272, notifier=w273) -> ()  [unwired: 1 in, 2 out]
                }
              }
              n166 = Select(t=Quick_Stack_Marked_Areas_Actions."Reset Path", s=w259, f=Quick_Stack_Marked_Areas_Actions."Switch") -> (s? t:f=w268:T3)
            }
            frame "Switch" {
              n167 = property on="Marked Positions" class="MCListbox (strict)"() -> ("Value"=w308:i32)  [unwired: 2 in, 2 out]
              n168 = Array Size(array=w304) -> (size(s)=w307:i32)
              n169 = Increment(x=w308) -> (x+1=w303:i32)
              n170 = Greater Or Equal?(x=w303, y=w307) -> (x >= y?=w297:bool)
              n171 = case shown="True" w297 {
                tunnel: w303 -> [w311 _]
                tunnel: [w311 0] -> w302
                tunnel: w301 -> [w310 w313]
                tunnel: [w310 w312] -> w299
                frame False {
                }
                frame True {
                  n172 = Increment(x=w313) -> (x+1=w312:u16)
                }
              }
              n173 = Equal?(x="Number of Cycles", y=w299) -> (x = y?=w298:bool)
              n174 = property on="Marked Positions" class="MCListbox (strict)"("Value"=w302) -> ()  [unwired: 2 in, 2 out]
              n175 = Implies(1:w298, 2:w297) -> (0:w294:bool)
              n176 = Select(t=Quick_Stack_Marked_Areas_Actions."Move to Position" ("y"), s=w294, f=Quick_Stack_Marked_Areas_Actions."Delay" ("y")) -> (s? t:f=w293:T3)
              n177 = Select(t=Quick_Stack_Marked_Areas_Actions."Reset Path" ("y"), s=w298, f=w293) -> (s? t:f=w305:T3)
            }
            frame "Delay" {
              n178 = Multiply(x="Cycle Delay (s)", y=u32 10) -> (x*y=w325:u32)
              n179 = To Long Integer(number=w325) -> (32bit integer=w326:i32)
              n180 = for {
                N: w326 -> [_]
                tunnel: w320 -> [w338]
                tunnel: [w336] -> w319
                tunnel: w318 -> [w331]
                tunnel: [w331] -> w317
                i -> [w335]
                stop <- w336 stop-if-true
                n181 = To Double Precision Float(number=w335) -> (double precision float=w334:dbl)
                n182 = Get Notifier Status(notifier=w338) -> (current notification=w337:T3)  [unwired: 1 in, 4 out]
                n183 = Equal?(x=w337, y=Quick_Stack_Marked_Areas_Actions."Abort") -> (x = y?=w336:bool)
                n184 = Divide(x=w334, y=10.0) -> (x/y=→"Current Delay Time (s)":dbl)
                n185 = Wait (ms)(milliseconds to wait=u32 100) -> ()  [unwired: 1 out]
              }
              n186 = Increment(x=w317) -> (x+1=→"Current Cycle":u16)
              n187 = Select(t=Quick_Stack_Marked_Areas_Actions."Reset Path" ("y"), s=w319, f=Quick_Stack_Marked_Areas_Actions."Move to Position" ("y")) -> (s? t:f=w321:T3)
            }
            frame "Reset Path" {
              n188 = Get Notifier Status(notifier=w346) -> (notifier out=w345:refnum<notifier>, current notification=w344:T1)  [unwired: 1 in, 3 out]
              n189 = Bundle By Name(cluster=w344, "Actions"=Quick_Stack_Actions."Idle", "Save Path"=w341) -> (w342:T1)
              n190 = Send Notification(notification=w342, notifier=w345) -> ()  [unwired: 1 in, 2 out]
            }
            frame "Remove Position" {
              n191 = property on="Marked Positions" class="MCListbox (strict)"() -> ("Value"=w355:i32)  [unwired: 2 in, 2 out]
              n192 = Delete From Array(array=w353, length=1, index=w355) -> (array with subset deleted=w352:T1[])  [unwired: 1 out]
            }
            frame "Clear All" {
            }
            frame "Quit" {
              n193 = Release Notifier(notifier=w367) -> ()  [unwired: 2 in, 3 out]
              n194 = Release Notifier(notifier=w366) -> ()  [unwired: 2 in, 3 out]
            }
          }
        }
      }
      n195 = local write "Quit"(w66) -> ()
    }
    frame Error {
    }
  }
  n196 = property class="VI"(reference=w14) -> (reference out=w23:refnum<vi>, "Panel"=w15:refnum<vi>)  [unwired: 1 in, 1 out]
  n197 = property class="Pnl"(reference=w15) -> ("Decos[]"=w13:refnum<vi>[], "Panes[]"=w19:refnum<vi>[])  [unwired: 1 in, 2 out]
  n198 = Array Size(array=w13) -> (size(s)=w11:i32)
  n199 = Decrement(x=w11) -> (x-1=w12:i32)
  n200 = Index Array(array=w19, index=0) -> (element=w18:refnum<vi>)
  n201 = Index Array(array=w13, index=w12) -> (element=w21:refnum<vi>)
  n202 = property class="VI"(reference=w23) -> (reference out=w25:refnum<vi>, "Front Panel.PanelBounds"=w26:T12)  [unwired: 1 in, 1 out]
  n203 = property class="Decor"(reference=w21) -> ("Bounds"=w24:T13)  [unwired: 1 in, 2 out]
  n204 = property class="Pane"(reference=w18, "Origin"=T5 {"Horizontal"=0, "Vertical"=0}, "HorizScrollbarVisibility"=w22, "VertScrollbarVisibility"=w22) -> ()  [unwired: 1 in, 2 out]
  n205 = Unbundle By Name(w24) -> ("Width"=w29:u32, "Height"=w32:u32)
  n206 = control-ref of="Quit"() -> (w16:refnum<vi>)
  n207 = To Word Integer(number=w29) -> (16bit integer=w31:i16)
  n208 = To Word Integer(number=w32) -> ()  [unwired: 1 out]
  n209 = property class="Bool (strict)"(reference=w16) -> ("Height"=w34:u32, "Top"=w35:i32)  [unwired: 1 in, 2 out]
  n210 = Unbundle By Name(w26) -> ("Left"=w28:i16, "Top"=w39:i16)
  n211 = To Word Integer(number=w34) -> (16bit integer=w37:i16)
  n212 = To Word Integer(number=w35) -> (16bit integer=w38:i16)
  n213 = Add(x=w28, y=w31) -> (x+y=w30:i16)
  n214 = Compound Arithmetic op=ADD(w39, w37, w38, i16 12 ("y")) -> (w33:i16)
  n215 = Bundle By Name(cluster=w26, "Right"=w30, "Bottom"=w33) -> (w27:T12)
  n216 = property class="VI"(reference=w25, "Front Panel.PanelBounds"=w27) -> ()  [unwired: 1 in, 2 out]
